vi "RT Main.vi"() -> ()   [LabVIEW 2018]
doc: "This VI will will initialize the FPGA VI and then stream analog input data from 4 channels of the 9203."
uses:
  <vilib>/Skyline/Tag/Shared/typedefs/DataType.ctl
  <vilib>/DAQmx/read.llb/DAQmx Read (Analog 1D Wfm NChan NSamp).vi
  <vilib>/DAQmx/write.llb/DAQmx Write (Analog 1D Wfm NChan NSamp).vi
  <vilib>/DAQmx/create/channels.llb/DAQmx Create Channel (AO-Voltage-Basic).vi
  <vilib>/DAQmx/configure/timing.llb/DAQmx Timing (Sample Clock).vi
  <vilib>/DAQmx/miscellaneous.llb/DAQmx Fill In Error Info.vi
  <vilib>/Skyline/Tag/Wrapper/Wrapper AMQP_class/Open Tag AMQP.vi
  <vilib>/Skyline/Tag/Wrapper/Wrapper_class/Write Tag (DBL).vi
  <vilib>/Skyline/Tag/Wrapper/Wrapper_class/Close Tag (Single).vi
  <vilib>/Skyline/Tag/Wrapper/Wrapper_class/Write Tag (Boolean).vi
  <vilib>/DAQmx/create/channels.llb/DAQmx Create Channel (AI-Voltage-Basic).vi
  <vilib>/FPGAPlugInAG/cRIO-9043/niLvFpga_Open_cRIO-9043.vi
  <vilib>/rvi/interface/common/dynamic/niFpgaDynamicAddResources.vi
  <vilib>/DAQmx/configure/trigger.llb/DAQmx Start Trigger (Time).vi
  <vilib>/Utility/error.llb/Error Cluster From Error Code.vi
  <vilib>/rvi/errors/niLvFpgaAdjustHostInterfaceError.vi
  <vilib>/FPGAPlugInAG/Dynamic/niLvFpga_Close_Dynamic.vi
  <vilib>/rvi/interface/nirviOpenFPGA/nirviOpenFPGA.xnode
  FPGA Bitfiles/NSRRCProject_NI 9215 TSN Sync(FP_IPNwjmrilpM.lvbitx
  NI 9215 TSN Sync(FPGA).vi
  <vilib>/rvi/interface/nirviReadWriteControl/nirviReadWriteControl.xnode
  <vilib>/rvi/interface/nirviMethod/nirviMethod.xnode
  <vilib>/rvi/interface/nirviCloseFPGA/nirviCloseFPGA.xnode
  <vilib>/rvi/interface/Simulation/niFpgaSimulationCallBeginRW.vi
  <vilib>/rvi/errors/niLvFpgaMergeErrorWithErrorCode.vi
  <resource>/objmgr/daqmx.rc
  <vilib>/measure/NI_MABase.lvlib
  NiFpgaLv.dll
  <vilib>/FPGAPlugInAG/Dynamic/niLvFpga_ReadFifo_Dynamic.vi
  <vilib>/Skyline/Tag/Wrapper/Wrapper_class/NI Skyline Tag.lvclass
  <vilib>/Skyline/Tag/Shared/NI Skyline Tag.lvlib
  <vilib>/Skyline/Tag/Wrapper/Wrapper AMQP_class/NI Skyline Tag AMQP.lvclass
panel:
  out "Time Delay (ns)":dbl(knob)=11.707899025873571 scale=0.0..200.0
  out "output cluster":cluster{"Fs":dbl, "#s":dbl}={"Fs"=10000.0, "#s"=2000.0}
  out "size(s)":i32=2000
  in  "AO Signal Type":T1(array[cluster])=[{"Waveform Type"=0, "Amplitude"=2.0, "Frequency"=500.0}] {"Frequency" format="%0.2p"; "Amplitude" format="%0.2p"; "Waveform Type" items=["Sine Wave", "Triangle Wave", "Square Wave", "Sawtooth Wave"]}
  in  "AO # of Samples":i32=2000
  in  "AO Sample Rate":dbl=10000.0
  in  "AO Channel":tag="Mod4/ao0"
  out "Actual AO S. Rate":dbl=10000.0 format="%0.2f"
  in  "AI Rate (Hz)":dbl=20000.0 format="%#.6p"
  out "Phase Histogram":T2(graph)={"X Values"=[0.7405687766790539, 2.2158941660011613, 3.6912195553232685, 5.166544944645376, 6.641870333967484, 8.11719572328959, 9.592521112611697, 11.067846501933804, 12.543171891255911, 14.018497280578018, 15.493822669900124, 16.96914805922223, 18.44447344854434, 19.91979883786645, 21.395124227188557, 22.870449616510665, 24.345775005832774, 25.821100395154883, 27.29642578447699, 28.7717511737991, 30.247076563121208, 31.722401952443317, 33.19772734176542, 34.67305273108753, 36.14837812040964, 37.62370350973175, 39.099028899053856, 40.574354288375964, 42.04967967769807, 43.52500506702018, 45.00033045634229, 46.4756558456644, 47.95098123498651, 49.426306624308616, 50.901632013630724, 52.37695740295283, 53.85228279227494, 55.32760818159705, 56.80293357091916, 58.27825896024127, 59.753584349563376, 61.228909738885484, 62.70423512820759, 64.1795605175297, 65.6548859068518, 67.13021129617391, 68.60553668549602, 70.08086207481813, 71.55618746414024, 73.03151285346235, 74.50683824278445, 75.98216363210656, 77.45748902142867, 78.93281441075078, 80.40813980007289, 81.883465189395, 83.3587905787171, 84.83411596803921, 86.30944135736132, 87.78476674668343, 89.26009213600554, 90.73541752532765, 92.21074291464976, 93.68606830397187, 95.16139369329397, 96.63671908261608, 98.11204447193819, 99.5873698612603, 101.06269525058241, 102.53802063990452, 104.01334602922662, 105.48867141854873, 106.96399680787084, 108.43932219719295, 109.91464758651506, 111.38997297583717, 112.86529836515928, 114.34062375448138, 115.8159491438035, 117.2912745331256, 118.76659992244771, 120.24192531176982, 121.71725070109193, 123.19257609041404, 124.66790147973614, 126.14322686905825, 127.61855225838036, 129.09387764770247, 130.56920303702458, 132.0445284263467, 133.5198538156688, 134.9951792049909, 136.470504594313, 137.94582998363512, 139.42115537295723, 140.89648076227934, 142.37180615160145, 143.84713154092356, 145.32245693024566, 146.79778231956777, 148.27310770888988, 149.748433098212, 151.2237584875341, 152.6990838768562, 154.17440926617832, 155.64973465550042, 157.12506004482253, 158.60038543414464, 160.07571082346675, 161.55103621278886, 163.02636160211097, 164.50168699143308, 165.97701238075518, 167.4523377700773, 168.9276631593994, 170.4029885487215, 171.87831393804362, 173.35363932736573, 174.82896471668784, 176.30429010600994, 177.77961549533205, 179.25494088465416, 180.73026627397627, 182.20559166329838, 183.6809170526205, 185.1562424419426, 186.6315678312647, 188.1068932205868, 189.58221860990892, 191.05754399923103, 192.53286938855314, 194.00819477787525, 195.48352016719736, 196.95884555651946, 198.43417094584157, 199.90949633516368, 201.3848217244858, 202.8601471138079, 204.33547250313, 205.81079789245211, 207.28612328177422, 208.76144867109633, 210.23677406041844, 211.71209944974055, 213.18742483906266, 214.66275022838477, 216.13807561770687, 217.61340100702898, 219.0887263963511, 220.5640517856732, 222.0393771749953, 223.51470256431742, 224.99002795363953, 226.46535334296163, 227.94067873228374, 229.41600412160585, 230.89132951092796, 232.36665490025007, 233.84198028957218, 235.3173056788943, 236.7926310682164, 238.2679564575385, 239.7432818468606, 241.21860723618272, 242.69393262550483, 244.16925801482694, 245.64458340414905, 247.11990879347115, 248.59523418279326, 250.07055957211537, 251.54588496143748, 253.0212103507596, 254.4965357400817, 255.9718611294038, 257.4471865187259, 258.922511908048, 260.39783729737013, 261.87316268669224, 263.34848807601435, 264.82381346533646, 266.29913885465857, 267.7744642439807, 269.2497896333028, 270.7251150226249, 272.200440411947, 273.6757658012691, 275.1510911905912, 276.6264165799133, 278.10174196923543, 279.57706735855754, 281.05239274787965, 282.52771813720176, 284.00304352652387, 285.478368915846, 286.9536943051681, 288.4290196944902, 289.9043450838123, 291.3796704731344, 292.8549958624565, 294.3303212517786], "Histogram: h(x)"=[62, 47, 63, 60, 62, 81, 64, 45, 46, 52, 55, 55, 41, 58, 54, 54, 51, 38, 36, 50, 30, 43, 40, 30, 28, 31, 31, 37, 21, 26, 23, 26, 30, 16, 22, 17, 14, 15, 21, 15, 26, 17, 17, 16, 11, 10, 13, 11, 8, 11, 11, 11, 4, 12, 2, 12, 8, 7, 7, 7, 5, 4, 5, 6, 7, 8, 8, 4, 5, 3, 4, 4, 2, 1, 6, 3, 4, 5, 4, 2, 6, 6, 8, 2, 3, 2, 2, 3, 2, 2, 0, 5, 2, 1, 1, 0, 2, 5, 1, 0, 2, 2, 2, 2, 3, 2, 1, 2, 0, 1, 3, 2, 3, 3, 0, 0, 0, 1, 1, 0, 1, 0, 0, 1, 0, 1, 1, 0, 0, 0, 0, 0, 1, 0, 0, 0, 0, 0, 0, 0, 0, 2, 1, 0, 0, 0, 0, 0, 2, 1, 0, 0, 1, 0, 0, 0, 0, 1, 0, 0, 0, 0, 0, 0, 0, 0, 0, 1, 1, 0, 0, 0, 0, 0, 0, 0, 0, 0, 0, 0, 0, 0, 0, 1, 0, 0, 0, 0, 0, 0, 0, 0, 0, 0, 0, 0, 0, 0, 0, 1]}
  out "Phase Offset":dbl[][](graph)=[[-11.707899025873571, -5.8264623139819305, 26.651557050522396, -8.197887033123441, 5.52465642564769, 44.5872398082737, 172.63389309798256, 136.20478130391922, 7.804789738429483, 5.247656757645093, -22.209414714900873, -19.349593565512684, -9.720784223538168, -26.828008938340922, 6.753336335757302, -10.482809371780636, -72.00009076351604, 12.855702060285907, 14.415730617303643, -10.042530920624454, -53.50445665793657, -46.98567631886145, 73.61913369675445, 22.960987600723914, 39.59996728976232, 13.41376326669651, -33.94326411798199, 209.362655935702, -13.280131658886964, 154.10438461984737, -19.372367863162815, -3.394584366640538, -104.20640526827073, 1.2047605230115142, -14.014411112645073, -8.372200846820437, 71.67268571116026, -17.782919157989618, 57.00675092182683, 9.285302369237714, -51.23564119170821, -40.950131578876125, 37.99080923524081, -55.444273809902576, -13.382935439233972, 8.14284544650181, -24.874755762770896, 56.50041871494676, 58.26182463653621, -18.835219596089683, 13.201383868599171, 21.23362156844895, 62.616706746095346, 5.860249733069063, -25.64897210081704, 42.10199459780329, -23.580344189855754, -12.280025599496687, -161.8570912419514, -3.862433945129569, 3.6618606608215796, -94.59228894637461, 38.98187119678183, -7.728860131439065, -58.19679199883386, -43.75447331800723, 33.81417813885046, 22.226252996504833, -2.9161197484161816, 31.21670826060793, -15.333109860561322, -62.41454391429437, 88.91884777934915, -18.39734032791583, 76.24512165504173, 62.562611751111355, -6.1330031678704415, -0.8807486165479831, -96.21699901781182, -24.800794788680765, -24.937352985342233, 9.869457766877522, 61.197636301488174, 98.58835512110986, -4.069321699470796, -77.79881073060282, 10.764211944377804, -16.032148719838617, 14.789678665649499, -26.5233674174953, 25.657009590030622, 55.86016259877938, -14.374928377531173, 22.599984220562206, -10.63349258369936, -21.586840839421356, 18.563108260586127, 33.26946869137726, 5.978072469754087, -46.95421961529532, -44.479487493104756], [11.707899025873571, 5.8264623139819305, 26.651557050522396, 8.197887033123441, 5.52465642564769, 44.5872398082737, 172.63389309798256, 136.20478130391922, 7.804789738429483, 5.247656757645093, 22.209414714900873, 19.349593565512684, 9.720784223538168, 26.828008938340922, 6.753336335757302, 10.482809371780636, 72.00009076351604, 12.855702060285907, 14.415730617303643, 10.042530920624454, 53.50445665793657, 46.98567631886145, 73.61913369675445, 22.960987600723914, 39.59996728976232, 13.41376326669651, 33.94326411798199, 209.362655935702, 13.280131658886964, 154.10438461984737, 19.372367863162815, 3.394584366640538, 104.20640526827073, 1.2047605230115142, 14.014411112645073, 8.372200846820437, 71.67268571116026, 17.782919157989618, 57.00675092182683, 9.285302369237714, 51.23564119170821, 40.950131578876125, 37.99080923524081, 55.444273809902576, 13.382935439233972, 8.14284544650181, 24.874755762770896, 56.50041871494676, 58.26182463653621, 18.835219596089683, 13.201383868599171, 21.23362156844895, 62.616706746095346, 5.860249733069063, 25.64897210081704, 42.10199459780329, 23.580344189855754, 12.280025599496687, 161.8570912419514, 3.862433945129569, 3.6618606608215796, 94.59228894637461, 38.98187119678183, 7.728860131439065, 58.19679199883386, 43.75447331800723, 33.81417813885046, 22.226252996504833, 2.9161197484161816, 31.21670826060793, 15.333109860561322, 62.41454391429437, 88.91884777934915, 18.39734032791583, 76.24512165504173, 62.562611751111355, 6.1330031678704415, 0.8807486165479831, 96.21699901781182, 24.800794788680765, 24.937352985342233, 9.869457766877522, 61.197636301488174, 98.58835512110986, 4.069321699470796, 77.79881073060282, 10.764211944377804, 16.032148719838617, 14.789678665649499, 26.5233674174953, 25.657009590030622, 55.86016259877938, 14.374928377531173, 22.599984220562206, 10.63349258369936, 21.586840839421356, 18.563108260586127, 33.26946869137726, 5.978072469754087, 46.95421961529532, 44.479487493104756]]
  in  "Offset":dbl(slide)=1.0381679389312977 scale=0.0..2.0
  out "Samples/Loop":dbl=2000.0
  out "AI Waveform":waveform(dbl)[](graph)=[{"t0"=timestamp(3621376962.9 s since 1904-01-01), "dt"=4.999999999999997e-05, "Y"=array[2000 elements], "attributes"=variant("NI_ChannelName"=variant(string "cDAQ9185Mod1/ai0"), "NI_UnitDescription"=variant(string "Volts"))}, {"t0"=timestamp(3621376962.9 s since 1904-01-01), "dt"=4.999999999999997e-05, "Y"=array[2000 elements], "attributes"=variant("NI_ChannelName"=variant(string "cDAQ9185Mod1/ai0"), "NI_UnitDescription"=variant(string "Volts"))}] caption="Waveform Graph"
  in  "cDAQ  Channel":tag="cDAQ9185Mod1/ai0"
  out "Actual AI Sample Rate":dbl=20000.0 format="%0.2f"
  out "DAQ error":errorcluster
  out "Data FIFO Full":bool
  out "Host Error out":errorcluster
  out "FPGA Error out":errorcluster
  in  "stop":bool
  # "Overview: Demonstrates cRIO and cDAQ measurement with TSN, and transfer Data to Host VI through EPICS\nRequirements: LabVIEW Full Development System, LV FPGA\nInstructions: \n1) Configure the Device Channel and Signal Setting.\n2) Run the VI\n3) Run EPICS Client (Host) VI"
  # "cRIO-9043 Mod1 AO Setting"
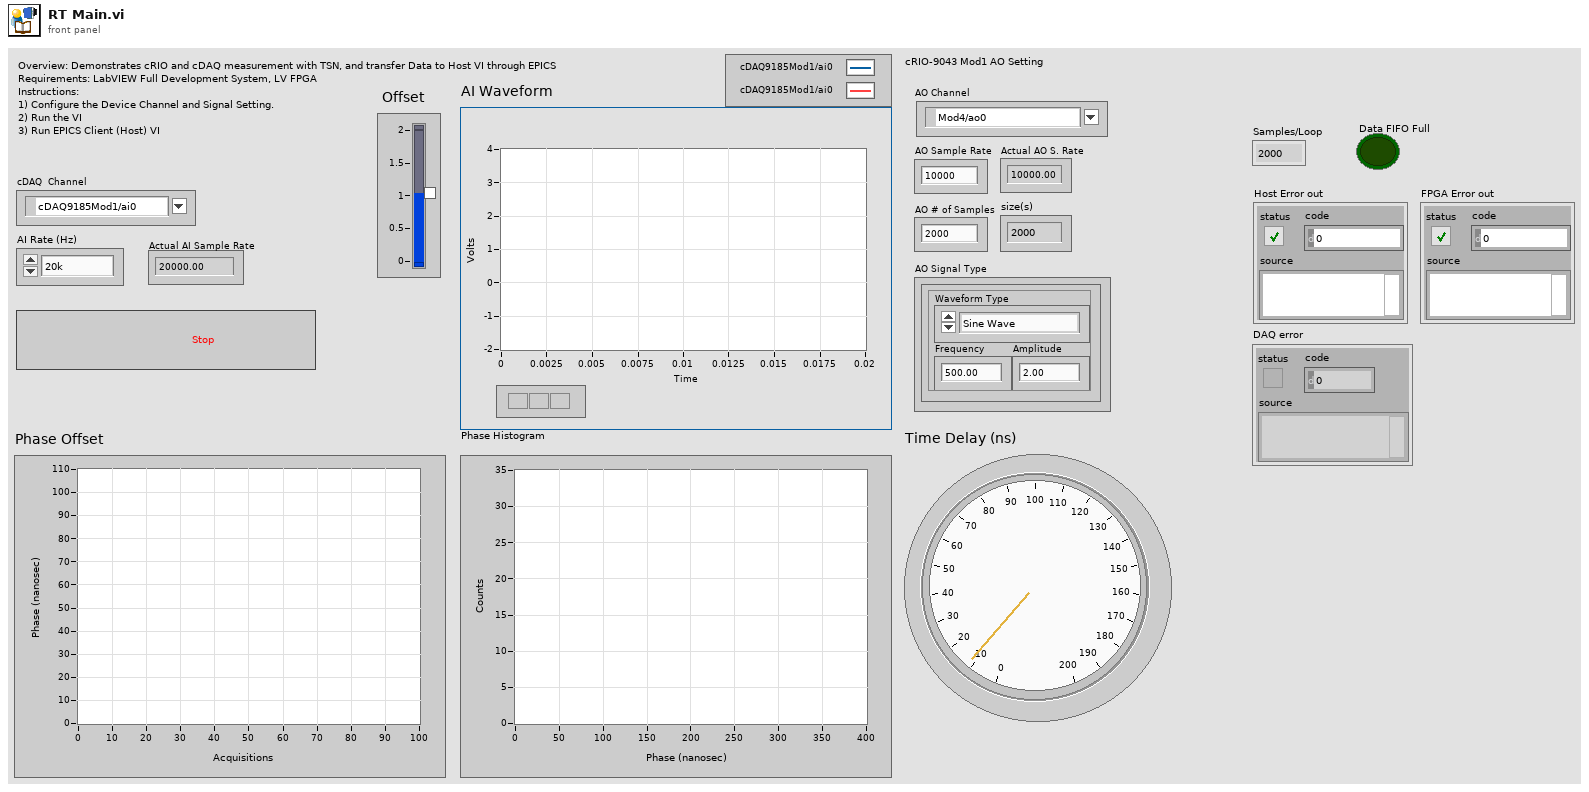
[diagram p1: front panel]
types:
  T1 = cluster{"Waveform Type":u16, "Amplitude":dbl, "Frequency":dbl}[]
  T2 = cluster{"X Values":dbl[], "Histogram: h(x)":i32[]}
  T3 = typedef "NI Skyline Tag.lvlib/DataType.ctl" = enum32{"Double", "I32", "String", "Boolean", "U64", "Timestamp"}
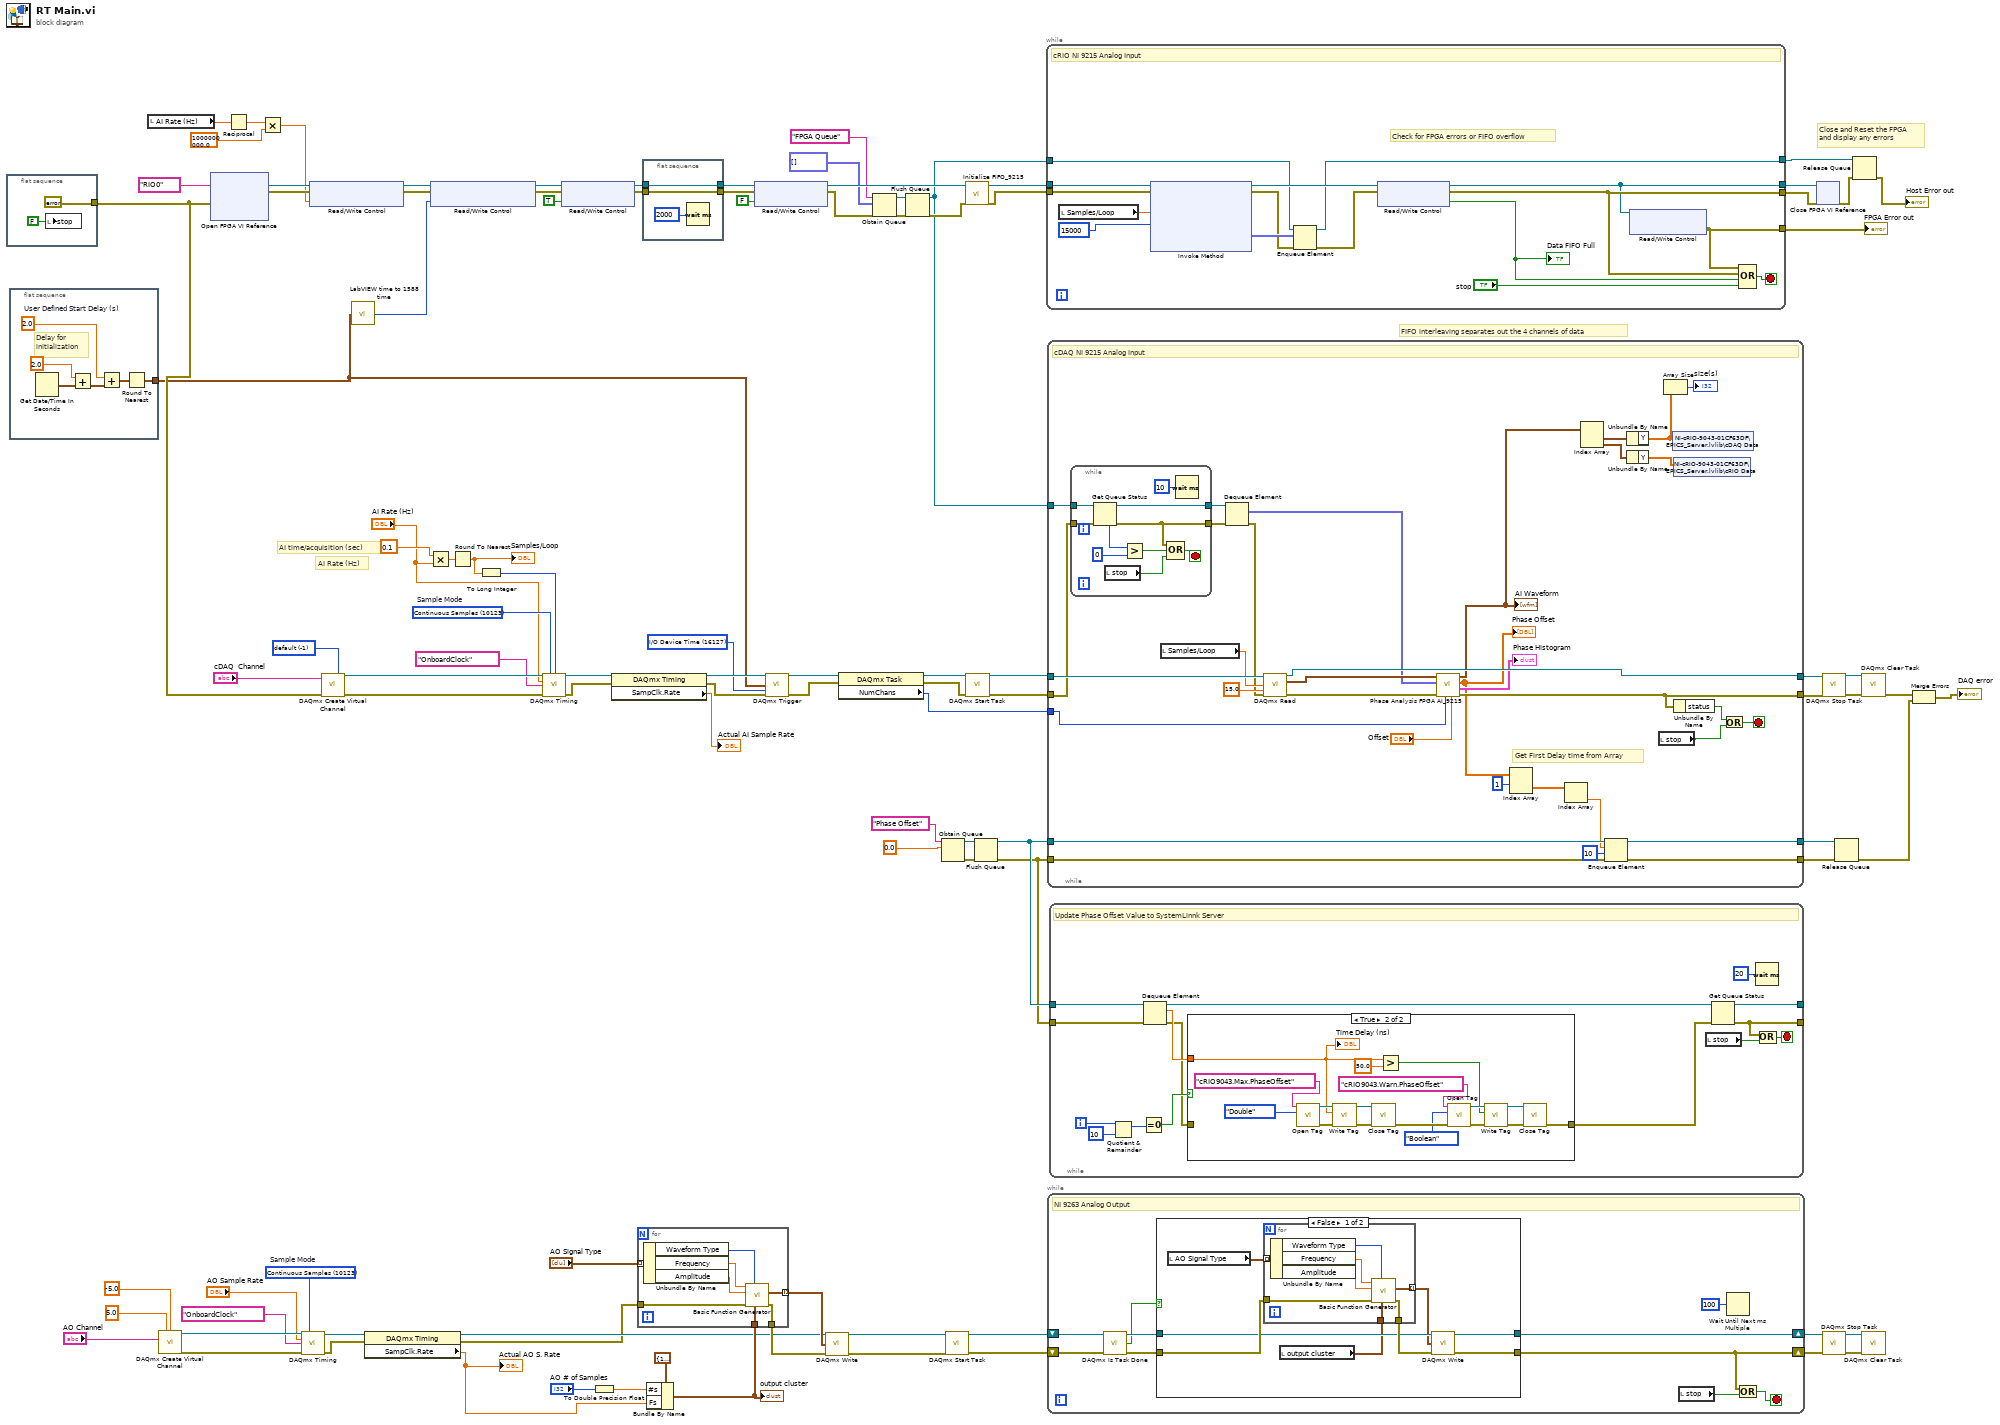
[diagram p0: block diagram]
diagram:
  w25 = 16127 items=["Host Time"=16126, "I/O Device Time"=16127] ("timescale")
  w60 = -1 items=["default"=-1, "RSE"=10083, "NRSE"=10078, "Differential"=10106, "Pseudodifferential"=12529] ("Terminal Configuration")
  w67 = 10123 items=["Finite Samples"=10178, "Continuous Samples"=10123, "Hardware Timed Single Point"=12522]  # Sample Mode
  w95 = 10123 items=["Finite Samples"=10178, "Continuous Samples"=10123, "Hardware Timed Single Point"=12522]  # Sample Mode
  # "AI Rate (Hz)"
  # "AI time/acquisition (sec)"
  # "Close and Reset the FPGA\nand display any errors"
  # "FIFO interleaving separates out the 4 channels of data"
  n1 = flat-sequence {
    tunnel: [errorcluster {"status"=FALSE, "code"=0, "source"=""} ("error in")] -> w34
    frame #0 {
      n2 = local write "stop"(FALSE ("stop")) -> ()
    }
  }
  n3 = flat-sequence {
    tunnel: [w110] -> w26
    frame #0 {
      w111 = 2.0  # User Defined Start Delay (s)
      # "Delay for\ninitialization"
      n4 = Get Date/Time In Seconds() -> (seconds since 1Jan1904=w109:timestamp)
      n5 = Add(x=2.0 ("Start Delay (s)"), y=w109) -> (x+y=w108:timestamp)
      n6 = Add(x=w111, y=w108) -> (x+y=w106:timestamp)
      n7 = Round To Nearest(number=w106) -> (nearest integer value=w110:timestamp)
    }
  }
  n8 = local read "AI Rate (Hz)"() -> (w15:dbl)
  n9 = call-poly <vilib>:"DAQmx Create Virtual Channel.vi"("maximum value"=5.0 ("Max Voltage"), "minimum value"=-5.0 ("Min Voltage"), "physical channels"="AO Channel") -> ("task out"=w93:refnum<k21>, "error out"=w94:errorcluster)  [unwired: 11 in]
  n10 = xnode "Open FPGA VI Reference"("error in"=w34, "resource name"=tag "RIO0") -> ("FPGA VI Reference Out"=w103:refnum<k20>, "error out"=w102:errorcluster)
  n11 = Reciprocal(x=w15) -> (1/x=w19:dbl)
  n12 = Multiply(x=w19, y=1000000000.0) -> (x*y=w17:dbl)
  n13 = call-poly <vilib>:"DAQmx Timing.vi"("task/channels in"=w93, "sample mode"=w95, "rate"="AO Sample Rate", "source"=tag "OnboardClock" ("Sample Clock Source"), "error in"=w94) -> ("task out"=w97:refnum<k21>, "error out"=w96:errorcluster)  [unwired: 9 in]
  n14 = xnode "Read/Write Control"("FPGA VI Reference In"=w103, "error in"=w102, "Sample Period (ns)"=w17) -> ("FPGA VI Reference Out"=w101:refnum<k20>, "error out"=w51:errorcluster)
  n15 = call-poly <vilib>:"DAQmx Create Virtual Channel.vi"("input terminal configuration"=w60, "physical channels"="cDAQ  Channel", "error in"=w34) -> ("task out"=w65:refnum<k21>, "error out"=w66:errorcluster)  [unwired: 11 in]
  n16 = call <userlib>:"LabVIEW time to 1588 time.vi"("labview time"=w26) -> ("1588 time in ns"=w36:u64)
  n17 = property class="DAQmx Timing"(reference=w97, error in=w96) -> (reference out=w77:refnum<k21>, error out=w76:errorcluster, "SampClk.Rate"=w86:dbl)
  "Actual AO S. Rate" <- w86
  n18 = Multiply(x=0.1 ("AI Acquisition Time (sec)"), y="AI Rate (Hz)") -> (x*y=w33:dbl)
  n19 = xnode "Read/Write Control"("FPGA VI Reference In"=w101, "error in"=w51, "Acquisition Start Time"=w36) -> ("FPGA VI Reference Out"=w53:refnum<k20>, "error out"=w52:errorcluster)
  n20 = Round To Nearest(number=w33) -> (nearest integer value=w31:dbl)
  "Samples/Loop" <- w31
  n21 = To Long Integer(number=w31) -> (32bit integer=w29:i32)
  n22 = call-poly <vilib>:"DAQmx Timing.vi"("task/channels in"=w65, "sample mode"=w67, "samples per channel"=w29, "rate"="AI Rate (Hz)", "source"=tag "OnboardClock" ("Sample Clock Source 2"), "error in"=w66) -> ("task out"=w69:refnum<k21>, "error out"=w68:errorcluster)  [unwired: 8 in]
  n23 = xnode "Read/Write Control"("FPGA VI Reference In"=w53, "error in"=w52, "Set Start Time"=TRUE) -> ("FPGA VI Reference Out"=w41:refnum<k20>, "error out"=w39:errorcluster)
  n24 = To Double Precision Float(number="AO # of Samples") -> (double precision float=w79:dbl)
  n25 = property class="DAQmx Timing"(reference=w69, error in=w68) -> (reference out=w54:refnum<k21>, error out=w27:errorcluster, "SampClk.Rate"=→"Actual AI Sample Rate":dbl)
  n26 = flat-sequence {
    tunnel: w41 -> [w114]
    tunnel: [w114] -> w40
    tunnel: w39 -> [w113]
    tunnel: [w113] -> w38
    frame #0 {
      n27 = Wait (ms)(milliseconds to wait=u32 2000) -> ()  [unwired: 1 out]
    }
  }
  n28 = Bundle By Name(cluster=cluster{"Fs":dbl, "#s":dbl} {"Fs"=1000.0, "#s"=1000.0} ("sampling info"), "#s"=w79, "Fs"=w86) -> (w85:cluster{"Fs":dbl, "#s":dbl})
  "output cluster" <- w85
  n29 = for {
    tunnel: w76 -> [w122]
    tunnel: w85 -> [w121]
    tunnel: [w120] -> w82
    tunnel: "AO Signal Type" -> [w119] mode=indexing
    tunnel: [w115] -> w80 mode=indexing
    n30 = Unbundle By Name(w119) -> ("Waveform Type"=w118:u16, "Frequency"=w117:dbl, "Amplitude"=w116:dbl)
    n31 = call <vilib>:"Basic Function Generator.vi"("sampling info"=w121, "signal type"=w118, "error in (no error)"=w122, "amplitude"=w116, "frequency"=w117) -> ("error out"=w120:errorcluster, "signal out"=w115:waveform(dbl))  [unwired: 4 in, 1 out]
  }
  n32 = xnode "Read/Write Control"("FPGA VI Reference In"=w40, "error in"=w38, "Set Start Time"=FALSE) -> ("FPGA VI Reference Out"=w50:refnum<k20>, "error out"=w44:errorcluster)
  n33 = call-poly <vilib>:"DAQmx Trigger.vi"("task/channels in"=w54, "when"=w26, "timescale"=w25, "error in"=w27) -> ("task out"=w28:refnum<k21>, "error out"=w23:errorcluster)  [unwired: 10 in]
  n34 = call-poly <vilib>:"DAQmx Write.vi"("task/channels in"=w77, "data"=w80, "error in"=w82) -> ("task out"=w84:refnum<k21>, "error out"=w83:errorcluster)  [unwired: 10 in, 1 out]
  n35 = property class="DAQmx Task"(reference=w28, error in=w23) -> (reference out=w24:refnum<k21>, error out=w22:errorcluster, "NumChans"=w21:u32)
  n36 = Obtain Queue(name (unnamed)="FPGA Queue", element data type=fxp<+/-,20,5>[] [] ("Data"), error in (no error)=w44) -> (queue out=w45:refnum<queue>, error out=w46:errorcluster)  [unwired: 2 in, 1 out]
  n37 = Flush Queue(queue=w45, error in (no error)=w46) -> (queue out=w20:refnum<queue>, error out=w47:errorcluster)  [unwired: 1 out]
  n38 = Obtain Queue(name (unnamed)="Phase Offset", element data type=0.0 ("mean")) -> (queue out=w12:refnum<queue>, error out=w11:errorcluster)  [unwired: 3 in, 1 out]
  n39 = call <vilib>:"DAQmx Start Task.vi"("task/channels in"=w84, "error in"=w83) -> ("task out"=w73:refnum<k21>, "error out"=w72:errorcluster)  [unwired: 12 in]
  n40 = call "Initialize FIFO_9215.vi"("error in (no error)"=w47, "FPGA Refnum Input"=w50) -> ("error out"=w48:errorcluster, "FPGA Refnum Output"=w49:refnum<k20>)  [unwired: 8 in]
  n41 = call <vilib>:"DAQmx Start Task.vi"("task/channels in"=w24, "error in"=w22) -> ("task out"=w64:refnum<k21>, "error out"=w63:errorcluster)  [unwired: 12 in]
  n42 = Flush Queue(queue=w12, error in (no error)=w11) -> (queue out=w3:refnum<queue>, error out=w2:errorcluster)  [unwired: 1 out]
  n43 = while {
    tunnel: w49 -> [w136]
    tunnel: w48 -> [w135]
    tunnel: [w131] -> w100
    tunnel: [w130] -> w99
    tunnel: [w129] -> w98
    tunnel: w20 -> [w124]
    tunnel: [w123] -> w10
    stop <- w133 stop-if-true
    # "Check for FPGA errors or FIFO overflow"
    # "cRIO NI 9215 Analog Input"
    n44 = local read "Samples/Loop"() -> (w128:dbl)
    n45 = xnode "Invoke Method"("FPGA VI Reference In"=w136, "error in"=w135, "Number of Elements"=w128, "Timeout (ms)"=15000) -> ("FPGA VI Reference Out"=w134:refnum<k20>, "error out"=w126:errorcluster, "Data"=w127:fxp<+/-,20,5>[])  [unwired: 1 out]
    n46 = Enqueue Element(queue=w124, element=w127, error in (no error)=w126) -> (queue out=w123:refnum<queue>, error out=w125:errorcluster)  [unwired: 1 in, 1 out]
    n47 = xnode "Read/Write Control"("FPGA VI Reference In"=w134, "error in"=w125) -> ("FPGA VI Reference Out"=w130:refnum<k20>, "error out"=w131:errorcluster, "Data FIFO Full"=w132:bool)
    "Data FIFO Full" <- w132
    n48 = xnode "Read/Write Control"("FPGA VI Reference In"=w130) -> ("FPGA Error Out"=w129:errorcluster)  [unwired: 1 in, 2 out]
    n49 = Compound Arithmetic op=OR(w129, w131, w132, "stop") -> (w133:bool)
  }
  "FPGA Error out" <- w98
  n50 = while {
    tunnel: w64 -> [w172]
    tunnel: w63 -> [w164]
    tunnel: [w171] -> w58
    tunnel: [w159] -> w57
    tunnel: w21 -> [w156]
    tunnel: w20 -> [w165]
    tunnel: w3 -> [w146]
    tunnel: w2 -> [w145]
    tunnel: [w144] -> w7
    tunnel: [w143] -> w6
    stop <- w169 stop-if-true
    # "Get First Delay time from Array"
    # "cDAQ NI 9215 Analog Input"
    n51 = while {
      tunnel: w164 -> [w182]
      tunnel: [w180] -> w163
      tunnel: [w173] -> w162
      tunnel: w165 -> [w176]
      stop <- w179 stop-if-true
      n52 = Get Queue Status(queue=w176, error in (no error)=w182) -> (queue out=w180:refnum<queue>, error out=w173:errorcluster, # elements in queue=w178:i32)  [unwired: 1 in, 5 out]
      n53 = local read "stop"() -> (w175:bool)
      n54 = Greater?(x=w178, y=0) -> (0:w174:bool)
      n55 = Compound Arithmetic op=OR(w173, w174, w175) -> (w179:bool)
      n56 = Wait (ms)(milliseconds to wait=u32 10) -> ()  [unwired: 1 out]
    }
    n57 = local read "Samples/Loop"() -> (w167:dbl)
    n58 = Dequeue Element(queue=w163, error in (no error)=w162) -> (element=w157:fxp<+/-,20,5>[], error out=w161:errorcluster)  [unwired: 1 in, 2 out]
    n59 = call-poly <vilib>:"DAQmx Read.vi"("task/channels in"=w172, "number of samples per channel"=w167, "timeout"=15.0, "error in"=w161) -> ("task out"=w171:refnum<k21>, "data"=w158:waveform(dbl)[], "error out"=w160:errorcluster)  [unwired: 9 in]
    n60 = call "Phase Analysis FPGA AI_9215.vi"("Offset"="Offset", "NumAI Channels"=w156, "error in (no error)"=w160, "LVFPGA Data in"=w157, "cDAQ data in"=w158) -> ("error out"=w159:errorcluster, "Phase Histogram"=→"Phase Histogram":T2, "Phase Plot"=w147:dbl[][], "Waveform Plot"=w153:waveform(dbl)[])  [unwired: 1 in, 2 out]
    "AI Waveform" <- w153
    "Phase Offset" <- w147
    n61 = Index Array(array=w147, index (row)=1) -> (element=w141:dbl[])  [unwired: 1 in]
    n62 = Index Array(array=w141) -> (element=w140:dbl)  [unwired: 1 in]
    n63 = Index Array(array=w153) -> (element #1=w152:waveform(dbl), element #2=w151:waveform(dbl))  [unwired: 2 in]
    n64 = Enqueue Element(queue=w146, element=w140, timeout in ms (-1)=10, error in (no error)=w145) -> (queue out=w144:refnum<queue>, error out=w143:errorcluster)  [unwired: 1 out]
    n65 = Unbundle By Name(w152) -> ("Y"=w150:dbl[])
    n66 = Unbundle By Name(w151) -> ("Y"=w148:dbl[])
    n67 = local read "stop"() -> (w168:bool)
    n68 = Array Size(array=w150) -> (size(s)=→"size(s)":i32)
    n69 = shared-variable "NI-cRIO-9043-01CF63DF\\EPICS_Server.lvlib\\cDAQ Data"(w150) -> ()  [unwired: 1 in, 1 out]
    n70 = shared-variable "NI-cRIO-9043-01CF63DF\\EPICS_Server.lvlib\\cRIO Data"(w148) -> ()  [unwired: 1 in, 1 out]
    n71 = Unbundle By Name(w159) -> ("status"=w170:bool)
    n72 = Or(x=w170, y=w168) -> (x .or. y?=w169:bool)
  }
  n73 = while {
    shift-right: [w185] -> w71
    shift-left: w73 -> [w192]
    shift-right: [w184] -> w70
    shift-left: w72 -> [w191]
    stop <- w190 stop-if-true
    # "NI 9263 Analog Output"
    n74 = call <vilib>:"DAQmx Is Task Done.vi"("task/channels in"=w192, "error in"=w191) -> ("task out"=w186:refnum<k21>, "task done?"=w183:bool, "error out"=w187:errorcluster)  [unwired: 11 in]
    n75 = case shown="False" w183 {
      tunnel: w187 -> [w198 w209]
      tunnel: w186 -> [w197 w210]
      tunnel: [w195 w210] -> w185
      tunnel: [w194 w209] -> w184
      frame False {
        n76 = local read "AO Signal Type"() -> (w200:T1)
        n77 = local read "output cluster"() -> (w196:cluster{"Fs":dbl, "#s":dbl})
        n78 = for {
          tunnel: w198 -> [w208]
          tunnel: w196 -> [w207]
          tunnel: [w206] -> w199
          tunnel: w200 -> [w205] mode=indexing
          tunnel: [w201] -> w193 mode=indexing
          n79 = Unbundle By Name(w205) -> ("Waveform Type"=w204:u16, "Frequency"=w203:dbl, "Amplitude"=w202:dbl)
          n80 = call <vilib>:"Basic Function Generator.vi"("sampling info"=w207, "signal type"=w204, "error in (no error)"=w208, "amplitude"=w202, "frequency"=w203) -> ("error out"=w206:errorcluster, "signal out"=w201:waveform(dbl))  [unwired: 4 in, 1 out]
        }
        n81 = call-poly <vilib>:"DAQmx Write.vi"("task/channels in"=w197, "data"=w193, "error in"=w199) -> ("task out"=w195:refnum<k21>, "error out"=w194:errorcluster)  [unwired: 10 in, 1 out]
      }
      frame True {
      }
    }
    n82 = local read "stop"() -> (w189:bool)
    n83 = Wait Until Next ms Multiple(millisecond multiple=u32 100) -> ()  [unwired: 1 out]
    n84 = Compound Arithmetic op=OR(w184, w189) -> (w190:bool)
  }
  n85 = while {
    tunnel: w3 -> [w225]
    tunnel: w2 -> [w223]
    tunnel: [w213] -> _
    tunnel: [w211] -> _
    i -> [w219]
    stop <- w220 stop-if-true
    # "Update Phase Offset Value to SystemLinnk Server"
    n86 = Quotient & Remainder(x=w219, y=10) -> (x-y*floor(x/y)=w217:i32)  [unwired: 1 out]
    n87 = Equal To 0?(x=w217) -> (x = 0?=w216:bool)
    n88 = Dequeue Element(queue=w225, error in (no error)=w223) -> (queue out=w222:refnum<queue>, element=w215:dbl, error out=w214:errorcluster)  [unwired: 1 in, 1 out]
    n89 = case shown="True" w216 {
      tunnel: w215 -> [_ w227]
      tunnel: w214 -> [w226 _]
      tunnel: [w226 w232] -> w212
      frame False {
      }
      frame True {
        n90 = call-poly <vilib>:"Open Tag.vi"("data type"=DataType."Double" ("Data Type"), "path"="cRIO9043.Max.PhaseOffset" ("Tag Path (Write)")) -> ("error out"=w243:errorcluster, "tag out"=w242:refnum<class "NI Skyline Tag.lvclass">)  [unwired: 8 in]
        n91 = call-poly <vilib>:"Write Tag.vi"("error in (no error)"=w243, "value"=w227, "tag in"=w242) -> ("error out"=w240:errorcluster, "tag out"=w241:refnum<class "NI Skyline Tag.lvclass">)  [unwired: 7 in]
        n92 = call-poly <vilib>:"Close Tag.vi"("error in (no error)"=w240, "tag in"=w241) -> ("error out"=w233:errorcluster)  [unwired: 9 in]
        n93 = Greater?(x=w227, y=50.0) -> (0:w228:bool)
        n94 = call-poly <vilib>:"Open Tag.vi"("error in (no error)"=w233, "data type"=DataType."Boolean", "path"="cRIO9043.Warn.PhaseOffset" ("Tag Path (Write)")) -> ("error out"=w237:errorcluster, "tag out"=w236:refnum<class "NI Skyline Tag.lvclass">)  [unwired: 7 in]
        n95 = call-poly <vilib>:"Write Tag.vi"("error in (no error)"=w237, "value"=w228, "tag in"=w236) -> ("error out"=w234:errorcluster, "tag out"=w235:refnum<class "NI Skyline Tag.lvclass">)  [unwired: 7 in]
        n96 = call-poly <vilib>:"Close Tag.vi"("error in (no error)"=w234, "tag in"=w235) -> ("error out"=w232:errorcluster)  [unwired: 9 in]
        "Time Delay (ns)" <- w227
      }
    }
    n97 = local read "stop"() -> (w221:bool)
    n98 = Get Queue Status(queue=w222, error in (no error)=w212) -> (queue out=w213:refnum<queue>, error out=w211:errorcluster)  [unwired: 1 in, 6 out]
    n99 = Wait (ms)(milliseconds to wait=u32 20) -> ()  [unwired: 1 out]
    n100 = Compound Arithmetic op=OR(w211, w221) -> (w220:bool)
  }
  n101 = xnode "Close FPGA VI Reference"("FPGA VI Reference In"=w99, "error in"=w100) -> ("error out"=w9:errorcluster)
  n102 = call <vilib>:"DAQmx Stop Task.vi"("task/channels in"=w58, "error in"=w57) -> ("task out"=w55:refnum<k21>, "error out"=w56:errorcluster)  [unwired: 12 in]
  n103 = call <vilib>:"DAQmx Stop Task.vi"("task/channels in"=w71, "error in"=w70) -> ("task out"=w75:refnum<k21>, "error out"=w74:errorcluster)  [unwired: 12 in]
  n104 = Release Queue(queue=w7, error in (no error)=w6) -> (error out=w4:errorcluster)  [unwired: 1 in, 2 out]
  n105 = Release Queue(queue=w10, error in (no error)=w9) -> (error out=→"Host Error out":errorcluster)  [unwired: 1 in, 2 out]
  n106 = call <vilib>:"DAQmx Clear Task.vi"("task in"=w55, "error in"=w56) -> ("error out"=w14:errorcluster)  [unwired: 13 in]
  n107 = call <vilib>:"DAQmx Clear Task.vi"("task in"=w75, "error in"=w74) -> ()  [unwired: 13 in, 1 out]
  n108 = Merge Errors(w14, w4) -> (→"DAQ error":errorcluster)
